vi "Resize.Calculate Pane Position and Size.vi"(4 "Origin for X,Y Max (Top Left)":T1(ring), 5 "Input Units (All Pixels)":u16(ring) items=["All Pixels"=0, "Left in Percent"=1, "Top in Percent"=2, "Right in Percent"=4, "Bottom in Percent"=8, "All Percent"=15], 6 "Origin for X,Y (Top Left)":T1(ring), 7 "Pane in":refnum<vi>, 8 "Y Max":dbl, 9 "X Max":dbl, 10 "Y Origin":dbl, 11 "X Origin":dbl) -> (2 "Size":cluster{u32, u32}, 3 "Position":cluster{"X Coordinate":i32, "Y Coordinate":i32})   [LabVIEW 2024, in "EQMF.lvlib" / "Controls.lvlib"]
uses:
  Controls.lvlib
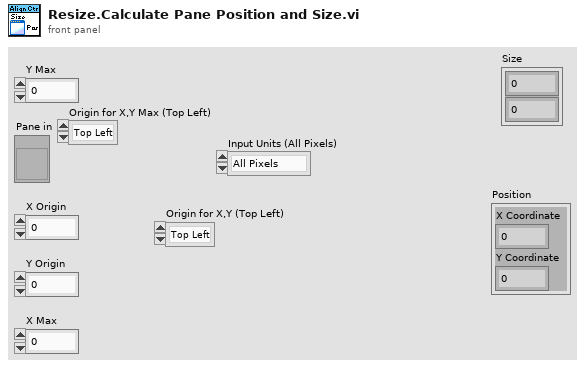
[diagram p1: front panel]
types:
  T1 = enum16{"Top Left", "Bottom Right", "Top Right", "Bottom Left"}
  T2 = cluster{"Screen X Coordinate":dbl, "Screen Y Coordinate":dbl}
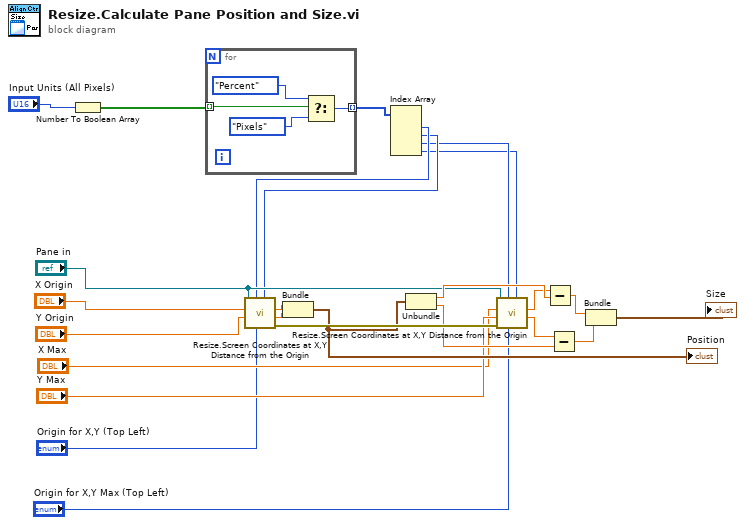
[diagram p0: block diagram]
diagram:
  n1 = Number To Boolean Array(number="Input Units (All Pixels)") -> (Boolean array=w8:bool[])
  n2 = for {
    tunnel: w8 -> [w29] mode=indexing
    tunnel: [w28] -> w7 mode=indexing
    n3 = Select(t=enum16{"Percent", "Pixels"}."Percent" ("X Units (Percent)"), s=w29, f=enum16{"Percent", "Pixels"}."Pixels" ("X Units (Percent)")) -> (s? t:f=w28:enum16{"Percent", "Pixels"})
  }
  n4 = Index Array(array=w7) -> (element #1=w6:enum16{"Percent", "Pixels"}, element #2=w5:enum16{"Percent", "Pixels"}, element #3=w4:enum16{"Percent", "Pixels"}, element #4=w3:enum16{"Percent", "Pixels"})  [unwired: 4 in]
  n5 = call "Resize.Screen Coordinates at X,Y Distance from the Origin.vi"("Y Units (Percent)"=w5, "Origin (Top Left)"="Origin for X,Y (Top Left)", "X Units (Percent)"=w6, "Y Distance"="Y Origin", "X Distance"="X Origin", "Pane Reference"="Pane in") -> ("error out"=w25:errorcluster, "Screen Y Coordinate"=w12:dbl, "Screen X Coordinate"=w11:dbl)  [unwired: 3 in]
  n6 = Bundle("Screen X Coordinate"=w11, "Screen Y Coordinate"=w12) -> (w17:T2)  [unwired: 1 in]
  "Position" <- w17
  n7 = Unbundle(w17) -> ("Screen X Coordinate"=w20:dbl, "Screen Y Coordinate"=w21:dbl)
  n8 = call "Resize.Screen Coordinates at X,Y Distance from the Origin.vi"("Y Units (Percent)"=w3, "Origin (Top Left)"="Origin for X,Y Max (Top Left)", "X Units (Percent)"=w4, "error in (no error)"=w25, "Y Distance"="Y Max", "X Distance"="X Max", "Pane Reference"="Pane in") -> ("Screen Y Coordinate"=w19:dbl, "Screen X Coordinate"=w18:dbl)  [unwired: 2 in, 1 out]
  n9 = Subtract(x=w18, y=w20) -> (x-y=w24:dbl)
  n10 = Subtract(x=w19, y=w21) -> (x-y=w23:dbl)
  n11 = Bundle(w24, w23) -> (→"Size":cluster{dbl, dbl})  [unwired: 1 in]
